vi "USB_CAN_VerInfo.vi"() -> (3 "VerInfo":string)   [LabVIEW 2011]
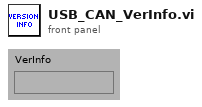
[diagram p1: front panel]
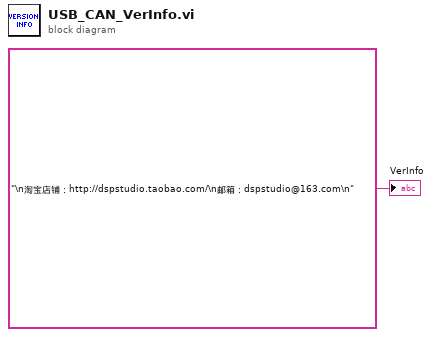
[diagram p0: block diagram]
diagram:
  "VerInfo" <- "\n淘宝店铺：http://dspstudio.taobao.com/\n邮箱：dspstudio@163.com\n" ("VerInfo")
